vi "FiberWLC_GenDistrs3.vi"(8 "Degeneracy 0->1":dbl, 9 "N4":u64, 10 "N8":u64) -> (2 "Degeneracy":dbl[](graph), 3 "ni":u32[][](graph))   [LabVIEW 2018]
uses:
  <vilib>/Analysis/1siggen.llb/Ramp Pattern by Samples.vi
  <vilib>/gmath/NI_Gmath.lvlib
  <vilib>/Analysis/NI_AALBase.lvlib
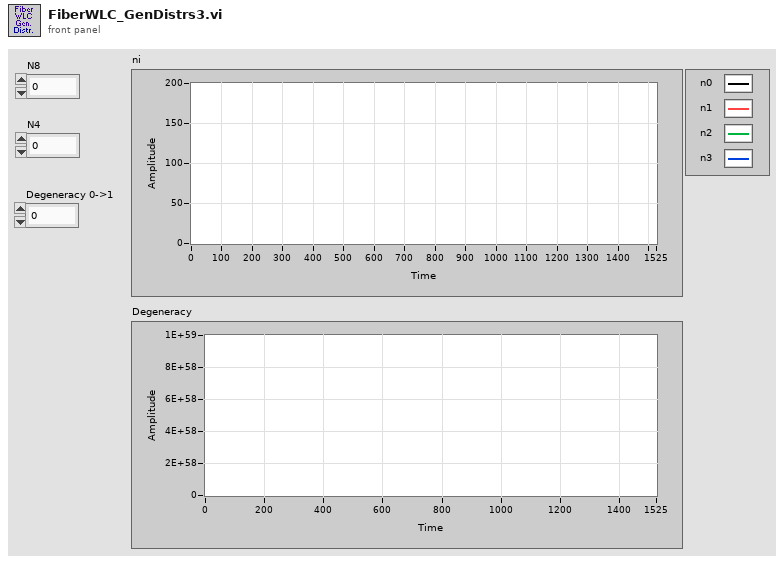
[diagram p1: front panel]
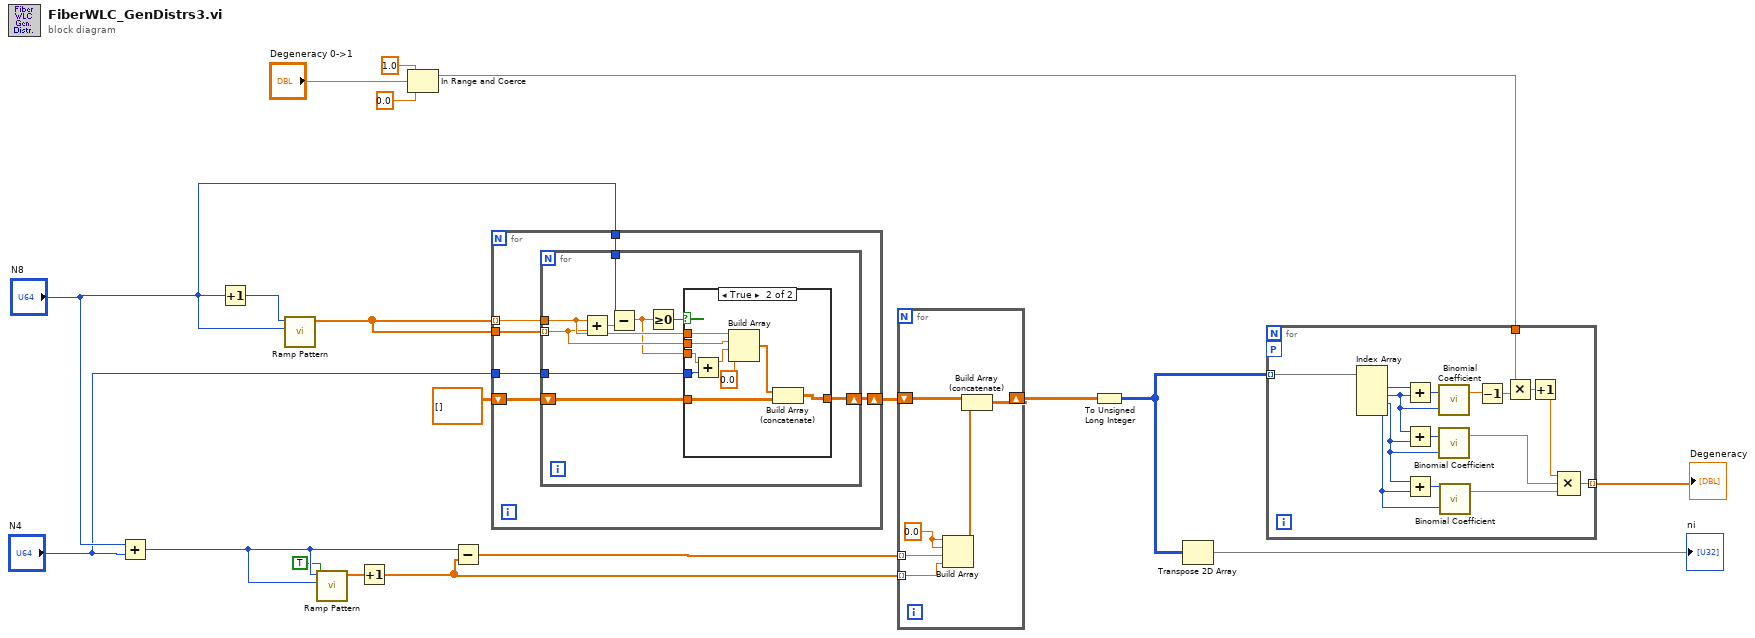
[diagram p0: block diagram]
diagram:
  n1 = Add(x="N8", y="N4") -> (x+y=w19:u64)
  n2 = Increment(x="N8") -> (x+1=w8:u64)
  n3 = call-poly <vilib>:"Ramp Pattern.vi"("end"="N8", "samples"=w8) -> ("Ramp Pattern"=w7:dbl[])  [unwired: 8 in, 1 out]
  n4 = call-poly <vilib>:"Ramp Pattern.vi"("exclude end?"=TRUE, "end"=w19, "samples"=w19) -> ("Ramp Pattern"=w5:dbl[])  [unwired: 7 in, 1 out]
  n5 = Increment(x=w5) -> (x+1=w3:dbl[])
  n6 = In Range and Coerce(upper limit=1.0, x="Degeneracy 0->1", lower limit=0.0) -> (coerced(x)=w13:dbl)  [unwired: 1 out]
  n7 = Subtract(x=w19, y=w3) -> (x-y=w2:dbl[])
  n8 = for {
    tunnel: w7 -> [w25] mode=indexing
    tunnel: w7 -> [w24]
    tunnel: "N8" -> [w23]
    shift-right: [w21] -> w1
    shift-left: dbl[][] [] -> [w22]
    tunnel: "N4" -> [w20]
    n9 = for {
      tunnel: w25 -> [w31]
      tunnel: w24 -> [w30] mode=indexing
      tunnel: w23 -> [w34]
      shift-right: [w27] -> w21
      shift-left: w22 -> [w28]
      tunnel: w20 -> [w26]
      n10 = Add(x=w31, y=w30) -> (x+y=w33:dbl)
      n11 = Subtract(x=w34, y=w33) -> (x-y=w29:dbl)
      n12 = Greater Or Equal To 0?(x=w29) -> (x >= 0?=w32:bool)
      n13 = case shown="True" w32 {
        tunnel: w31 -> [_ w44]
        tunnel: w30 -> [_ w43]
        tunnel: w29 -> [_ w42]
        tunnel: w28 -> [w35 w39]
        tunnel: [w35 w38] -> w27
        tunnel: w26 -> [_ w36]
        frame False {
        }
        frame True {
          n14 = Add(x=w42, y=w36) -> (x+y=w37:dbl)
          n15 = Build Array(w44, w43, w37, 0.0 ("element")) -> (w40:dbl[])
          n16 = Build Array (concatenate)(w40, w39) -> (w38:dbl[][])
        }
      }
    }
  }
  n17 = for {
    tunnel: w3 -> [w49] mode=indexing
    tunnel: w2 -> [w50] mode=indexing
    shift-right: [w45] -> w10
    shift-left: w1 -> [w47]
    w48 = 0.0 ("element")
    n18 = Build Array(w48, w48, w50, w49) -> (w46:dbl[])
    n19 = Build Array (concatenate)(w47, w46) -> (w45:dbl[][])
  }
  n20 = To Unsigned Long Integer(number=w10) -> (unsigned 32bit integer=w9:u32[][])
  n21 = Transpose 2D Array(2D array=w9) -> (transposed array=→"ni":u32[][])
  n22 = for {
    tunnel: w9 -> [w51] mode=indexing
    tunnel: w13 -> [w57]
    tunnel: [w52] -> w17 mode=indexing
    workers-P: _ -> [_]
    n23 = Index Array(array=w51) -> (element #1=w66:u32, element #2=w63:u32, element #3=w62:u32, element #4=w60:u32)  [unwired: 4 in]
    n24 = Add(x=w66, y=w63) -> (x+y=w65:u32)
    n25 = Add(x=w63, y=w62) -> (x+y=w64:u32)
    n26 = Add(x=w62, y=w60) -> (x+y=w61:u32)
    n27 = call <vilib>:"Binomial Coefficient.vi"("k"=w63, "n"=w65) -> ("binomial coefficient (n,k)"=w59:dbl)  [unwired: 1 out]
    n28 = call <vilib>:"Binomial Coefficient.vi"("k"=w62, "n"=w64) -> ("binomial coefficient (n,k)"=w54:dbl)  [unwired: 1 out]
    n29 = call <vilib>:"Binomial Coefficient.vi"("k"=w60, "n"=w61) -> ("binomial coefficient (n,k)"=w53:dbl)  [unwired: 1 out]
    n30 = Decrement(x=w59) -> (x-1=w56:dbl)
    n31 = Multiply(x=w57, y=w56) -> (x*y=w58:dbl)
    n32 = Increment(x=w58) -> (x+1=w55:dbl)
    n33 = Compound Arithmetic op=MULTIPLY(w55, w54, w53) -> (w52:dbl)
  }
  "Degeneracy" <- w17
